vi "Generic Camera Get Frame Num.vi"(0 "Image Ref":T1, 11 "Error In":errorcluster) -> (4 "Image Ref Dup":T1, 8 "Frame":u32, 15 "Error Out":errorcluster)   [LabVIEW 2025]
uses:
  <vilib>/vision/Image Controls.llb/IMAQ Image.ctl
  Camera Controls/Camera IMAQ Key Info.ctl
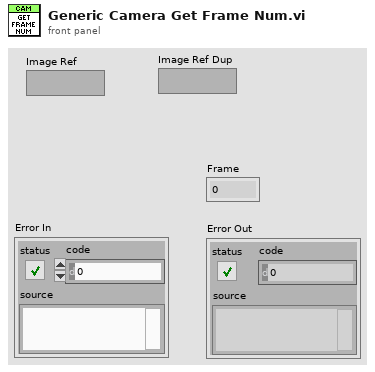
[diagram p1: front panel]
types:
  T1 = typedef "IMAQ Image.ctl" = refnum<image>
  T2 = typedef "Camera IMAQ Key Info.ctl" = cluster{"Frame":u32, "Sensor Height":i32, "Sensor Width":i32, "ROI Height":i32, "ROI Width":i32, "ROI Enable?":bool, "Bit per Pixel":u8}
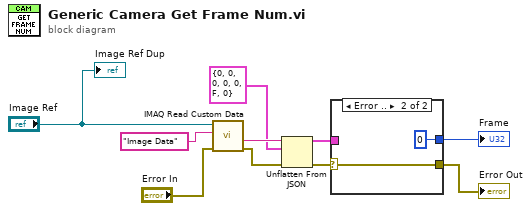
[diagram p0: block diagram]
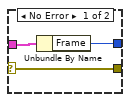
[diagram p2: hidden frame]
diagram:
  n1 = call "IMAQ Read Custom Data"("error in (no error)"="Error In", "Key"="Image Data", "Image"="Image Ref") -> ("error out"=w7:errorcluster, "Custom Data Out"=w8:string)  [unwired: 6 in, 1 out]
  n2 = Unflatten From JSON(JSON string=w8, type and defaults=T2 {"Frame"=0, "Sensor Height"=0, "Sensor Width"=0, "ROI Height"=0, "ROI Width"=0, "ROI Enable?"=FALSE, "Bit per Pixel"=0} ("Camera IMAQ Key Info"), error in (no error)=w7) -> (value=w3:T2, error out=w4:errorcluster)  [unwired: 4 in]
  n3 = case shown="Error .." w4 {
    selector: w4 -> [w11 w14]
    tunnel: w3 -> [w13 _]
    tunnel: [w12 u32 0 ("Frame")] -> w2
    tunnel: [w11 w14] -> w1
    frame No Error {
      n4 = Unbundle By Name(w13) -> ("Frame"=w12:u32)
    }
    frame Error {
    }
  }
  "Error Out" <- w1
  "Frame" <- w2
  "Image Ref Dup" <- "Image Ref"
